vi "Demo RGB LED - Chaser.vi"() -> ()   [LabVIEW 2015]
doc: "This example demonstrates a theater light chaser on a 1-wire RGB LED strip using a WS2811 or WS2812 controller. The color of all LEDs can be preset on the front panel as well as the number of lights to cycle in the light chase. The time delay can also be adjusted to change the dramatic effect."
uses:
  <vilib>/Aledyne-TSXperts/Arduino Compatible Compiler for LabVIEW/Code Generator/Arduino APIs/RGB LED Strip/RGB Strip Mode.ctl
  <vilib>/Aledyne-TSXperts/Arduino Compatible Compiler for LabVIEW/Arduino Compatible Compiler for LabVIEW.lvlib
panel:
  in  "delay (ms)":u8=25
  in  "Chase Every N Pixel":u8=2
  in  "Mode":T1 items=["400kHz_RGB"=0, "400kHz_GRB"=1, "400kHz_BRG"=4, "800kHz_RGB"=2, "800kHz_GRB"=3, "400kHz_BRG"=6]
  in  "Number of LEDs":u16=15
  in  "Blue":u8=127
  in  "Green":u8=127
  in  "Red":u8=127
  in  "Digital Pin":u8=13
  # "Overview: Demonstrates a theater light chaser on a 1-wire RGB LED strip using a WS2811 or WS2812 controller.  The color of all LEDs can be preset as well as the number of lights to cycle in the light chase.  The time delay can also be adjusted to change the dramatic effect.\n\nInstructions:\n1. Wire a 1-wire LED strip to a digital pin on the Arduino board.  Follow wiring instructions from the manufacturer.  A 100-500 ohm resistor is usually recommended between the Arduino digital output and the LED strip's data in pin.  Also, a 100 uF capacitor between the ground and power input may reduce noise on from the power supply.  It is also recommended to power the LED strip from a separate power input if available on the strip.  When daisy chaining LED strips, it is recommended to only daisy chain the Data line and to power each strip from a separate power input.\n2. Set the Digital Pin wired below.\n3. Set the Mode to the correct setting for your LED strip (the WS2812 uses 800kHz GRB).\n4. Set the Number of LEDs on your strip.  This can be set to any number equal to or smaller than the number of physical LEDs on the strip of you do not wish to power up all of them.\n5. Set Chase Every N Pixel to adjust how many pixels are moved on every cycle.\n6. Set the delay (ms) between LED rotations/shifts.\n7. Set the Red, Blue, and Green color of all LEDs on the strip.\n8.  If this example has been loaded from the Arduino Compatible Compiler for LabVIEW, simply select Compile and Download.  Otherwise, open Tools>Arduino Compatible Compiler for LabVIEW in LabVIEW, then select File>Load VI, and select this VI and then Compile and Download.\n9. Observe the LEDs on the strip as they appear to chase each other down the strip in a linear movement."
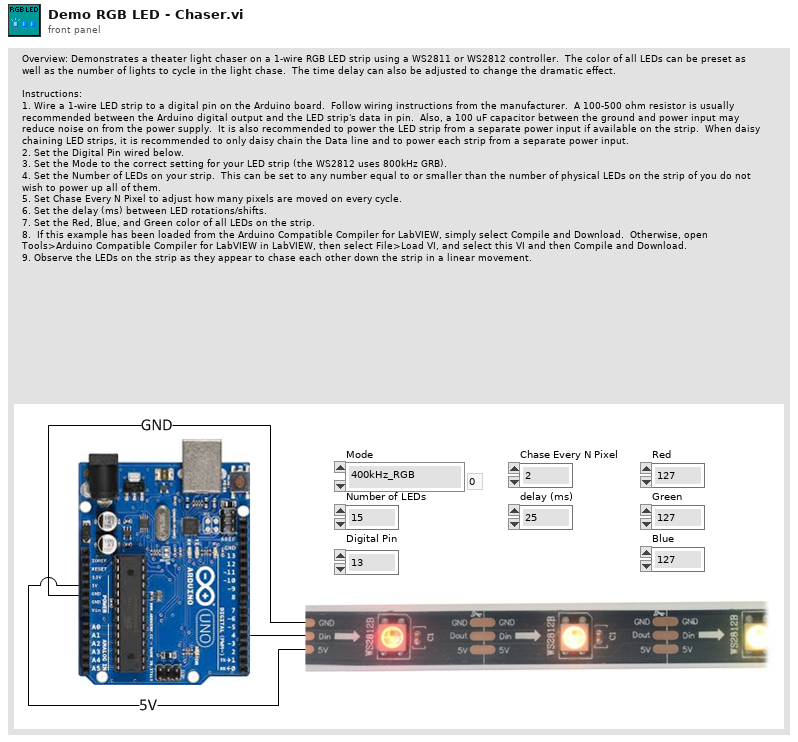
[diagram p1: front panel]
types:
  T1 = typedef "Arduino Compatible Compiler for LabVIEW.lvlib/RGB Strip Mode.ctl" = u16
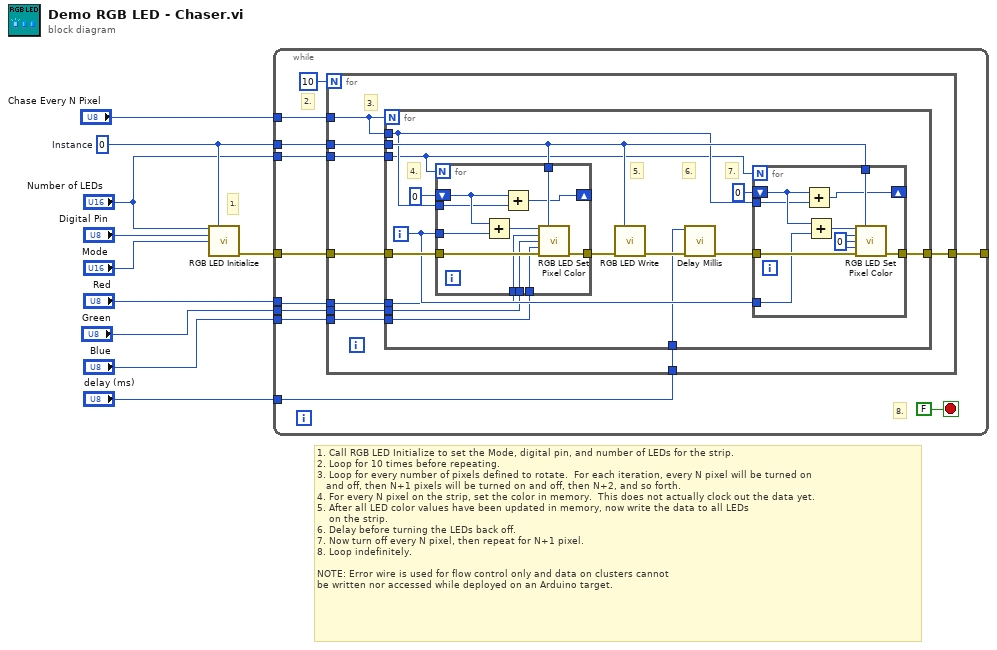
[diagram p0: block diagram]
diagram:
  w4 = u8 0  # Instance
  # "1."
  # "1. Call RGB LED Initialize to set the Mode, digital pin, and number of LEDs for the strip.\n2. Loop for 10 times before repeating.\n3. Loop for every number of pixels defined to rotate.  For each iteration, every N pixel will be turned on\n   and off, then N+1 pixels will be turned on and off, then N+2, and so forth.\n4. For every N pixel on the strip, set the color in memory.  This does not actually clock out the data yet. \n5. After all LED color values have been updated in memory, now write the data to all LEDs\n    on the strip.\n6. Delay before turning the LEDs back off.\n7. Now turn off every N pixel, then repeat for N+1 pixel.\n8. Loop indefinitely.\n\nNOTE: Error wire is used for flow control only and data on clusters cannot\nbe written nor accessed while deployed on an Arduino target."
  n1 = call <vilib>:"RGB LED Initialize.vi"("Number of Pixels"="Number of LEDs", "Instance"=w4, "Pin"="Digital Pin", "Mode"="Mode") -> ("error out"=w8:errorcluster)  [unwired: 11 in]
  n2 = while {
    tunnel: w8 -> [w19]
    tunnel: "Red" -> [w13]
    tunnel: "Green" -> [w12]
    tunnel: "Blue" -> [w11]
    tunnel: w4 -> [w18]
    tunnel: "Chase Every N Pixel" -> [w17]
    tunnel: "Number of LEDs" -> [w16]
    tunnel: [w15] -> _
    tunnel: "delay (ms)" -> [w14]
    stop <- FALSE stop-if-true
    # "8."
    # "2."
    n3 = for {
      N: u16 10 ("Number of Pixels") -> [_]
      tunnel: w18 -> [w30]
      tunnel: w19 -> [w29]
      tunnel: w17 -> [w28]
      tunnel: w16 -> [w27]
      tunnel: [w26] -> w15
      tunnel: w14 -> [w25]
      tunnel: w13 -> [w24]
      tunnel: w12 -> [w23]
      tunnel: w11 -> [w22]
      # "3."
      n4 = for {
        N: w28 -> [_]
        tunnel: w30 -> [w41]
        tunnel: w29 -> [w44]
        tunnel: w28 -> [w37]
        tunnel: w27 -> [w36]
        tunnel: [w35] -> w26
        tunnel: w25 -> [w34]
        tunnel: w24 -> [w33]
        tunnel: w23 -> [w32]
        tunnel: w22 -> [w31]
        i -> [w40]
        # "7."
        # "6."
        # "5."
        # "4."
        n5 = for {
          N: w36 -> [_]
          tunnel: w41 -> [w65]
          tunnel: w40 -> [w64]
          tunnel: [w63] -> w45
          tunnel: w44 -> [w62]
          shift-right: [w61] -> _
          shift-left: u8 0 ("Number of Pixels") -> [w59]
          tunnel: w37 -> [w58]
          tunnel: w33 -> [w57]
          tunnel: w32 -> [w56]
          tunnel: w31 -> [w55]
          n6 = Add(x=w59, y=w64) -> (x+y=w60:i32)
          n7 = Add(x=w59, y=w58) -> (x+y=w61:u8)
          n8 = call <vilib>:"RGB LED Set Pixel Color.vi"("Pixel"=w60, "Instance"=w65, "Red"=w57, "Green"=w56, "Blue"=w55, "error in (no error)"=w62) -> ("error out"=w63:errorcluster)  [unwired: 9 in]
        }
        n9 = call <vilib>:"RGB LED Write.vi"("Instance"=w41, "error in (no error)"=w45) -> ("error out"=w43:errorcluster)  [unwired: 13 in]
        n10 = call <vilib>:"Delay Millis.vi"("error in (no error)"=w43, "delay"=w34) -> ("error out"=w42:errorcluster)  [unwired: 9 in]
        n11 = for {
          N: w36 -> [_]
          tunnel: w41 -> [w54]
          tunnel: [w52] -> w35
          tunnel: w42 -> [w51]
          tunnel: w40 -> [w49]
          shift-right: [w48] -> _
          shift-left: u8 0 ("Number of Pixels") -> [w47]
          tunnel: w37 -> [w46]
          w50 = u8 0 ("Red")
          n12 = Add(x=w47, y=w46) -> (x+y=w48:u8)
          n13 = Add(x=w47, y=w49) -> (x+y=w53:i32)
          n14 = call <vilib>:"RGB LED Set Pixel Color.vi"("Pixel"=w53, "Instance"=w54, "Red"=w50, "Green"=w50, "Blue"=w50, "error in (no error)"=w51) -> ("error out"=w52:errorcluster)  [unwired: 9 in]
        }
      }
    }
  }
